vi "InitQueues.vi"() -> (0 "error out":errorcluster, 3 "QueueCluster":T1)   [LabVIEW 2017]
uses:
  CTRLS/EventCluster.ctl
  CTRLS/ListenMsg.ctl
  CTRLS/MainCluster.ctl
  MainMsg.ctl
  CTRLS/DAQCluster.ctl
  DaqMsg.ctl
  CTRLS/GUICluster.ctl
  CTRLS/GUIMsg.ctl
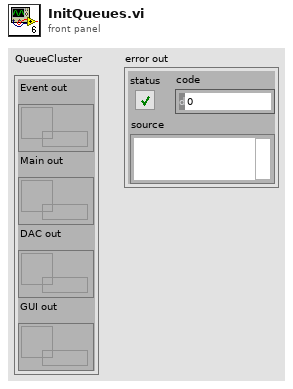
[diagram p1: front panel]
types:
  T1 = cluster{"Event out":refnum<queue>, "Main out":refnum<queue>, "DAC out":refnum<queue>, "GUI out":refnum<queue>}
  T2 = typedef "GUICluster.ctl" = cluster{"GUIMsg":T3, "GUINum":dbl, "GUIStr":string}
  T3 = typedef "GUIMsg.ctl" = enum16{"Init", "Halt", "WaterFlow", "AirFlow", "WaterPress", "AirPress", "WaterTemp", "NozzleForce", "SaveState", "MonState"}
  T4 = typedef "MainCluster.ctl" = cluster{"MainMsg":T5, "MainNum":dbl, "MainStr":string}
  T5 = typedef "MainMsg.ctl" = enum16{"Init", "Halt", "MonitorState", "SaveState", "Filename", "AirFlow", "WaterFlow", "AirPress", "WaterPress", "WaterTemp", "NozzleForce", "SaveAll", "Error", "Supervisor"}
  T6 = typedef "EventCluster.ctl" = cluster{"EventMsg":T7, "EventNum":dbl, "EventStr":string}
  T7 = typedef "ListenMsg.ctl" = enum16{"Init", "Halt", "Listen", "Error"}
  T8 = typedef "DAQCluster.ctl" = cluster{"DAQMsg":T9, "DAQNum":dbl, "DAQStr":string}
  T9 = typedef "DaqMsg.ctl" = enum16{"Init", "Halt", "GetMeasurement", "Stop", "Error"}
  T10 = cluster{"queue out":refnum<queue>, "queue out":refnum<queue>, "queue out":refnum<queue>, "queue out":refnum<queue>}
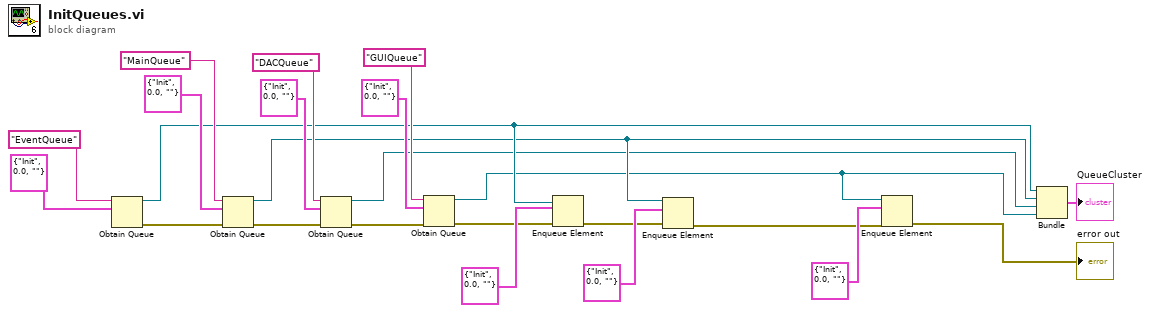
[diagram p0: block diagram]
diagram:
  n1 = Obtain Queue(name (unnamed)="EventQueue", element data type=T6 {"EventMsg"=enum."Init", "EventNum"=0.0, "EventStr"=""} ("EventCluster")) -> (queue out=w7:refnum<queue>, error out=w19:errorcluster)  [unwired: 3 in, 1 out]
  n2 = Obtain Queue(name (unnamed)="MainQueue", element data type=T4 {"MainMsg"=enum."Init", "MainNum"=0.0, "MainStr"=""} ("MainCluster"), error in (no error)=w19) -> (queue out=w6:refnum<queue>, error out=w18:errorcluster)  [unwired: 2 in, 1 out]
  n3 = Obtain Queue(name (unnamed)="DACQueue", element data type=T8 {"DAQMsg"=enum."Init", "DAQNum"=0.0, "DAQStr"=""} ("DAQCluster"), error in (no error)=w18) -> (queue out=w5:refnum<queue>, error out=w17:errorcluster)  [unwired: 2 in, 1 out]
  n4 = Obtain Queue(name (unnamed)="GUIQueue", element data type=T2 {"GUIMsg"=enum."Init", "GUINum"=0.0, "GUIStr"=""} ("GUICluster"), error in (no error)=w17) -> (queue out=w4:refnum<queue>, error out=w9:errorcluster)  [unwired: 2 in, 1 out]
  n5 = Enqueue Element(queue=w7, element=T6 {"EventMsg"=enum."Init", "EventNum"=0.0, "EventStr"=""}, error in (no error)=w9) -> (error out=w8:errorcluster)  [unwired: 1 in, 2 out]
  n6 = Enqueue Element(queue=w6, element=T4 {"MainMsg"=enum."Init", "MainNum"=0.0, "MainStr"=""}, error in (no error)=w8) -> (error out=w1:errorcluster)  [unwired: 1 in, 2 out]
  n7 = Enqueue Element(queue=w4, element=T2 {"GUIMsg"=enum."Init", "GUINum"=0.0, "GUIStr"=""}, error in (no error)=w1) -> (error out=→"error out":errorcluster)  [unwired: 1 in, 2 out]
  n8 = Bundle("queue out"=w7, "queue out"=w6, "queue out"=w5, "queue out"=w4) -> (→"QueueCluster":T10)  [unwired: 1 in]
